vi "midiInGetNumDevs.vi"(8 "error in":errorcluster, 11 "midi in":refnum<class "midi.lvclass">) -> (0 "error out":errorcluster, 2 "Number of MIDI Input Devices":i32, 3 "midi out":refnum<class "midi.lvclass">)   [LabVIEW 2020, in "midi.lvclass"]
doc: "The midiInGetNumDevs function retrieves the number of MIDI input devices in the system.\n\nReturns the number of MIDI input devices present in the system. A return value of zero means that there are no devices (not that there is no error)."
uses:
  midi.lvclass
  midi.lvclass/midi.ctl
  winmm.dll
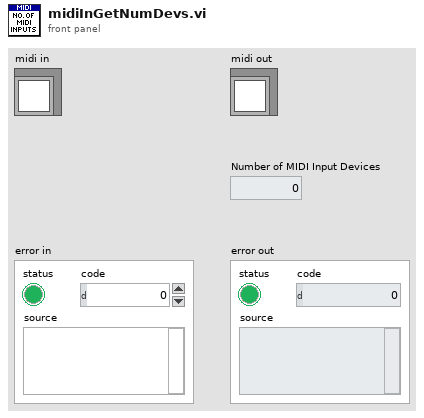
[diagram p1: front panel]
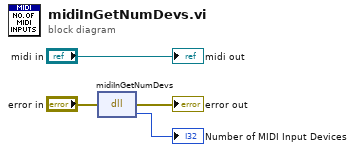
[diagram p0: block diagram]
diagram:
  n1 = dll-call lib="winmm.dll" fn="midiInGetNumDevs"(error in="error in") -> (error out=→"error out":errorcluster, "NumberOfInDevices"=→"Number of MIDI Input Devices":i32)  [unwired: 2 in, 1 out]
  "midi out" <- "midi in"
